vi "Timer Embedded.vi"(9 "Time Limit":u32, 10 "Reset":bool, 11 "Start Time In":u32) -> (2 "Time Limit Passed":bool, 3 "Start Time Out":u32)   [LabVIEW 2015]
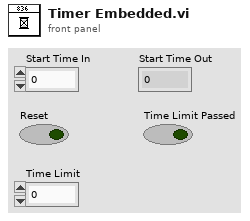
[diagram p1: front panel]
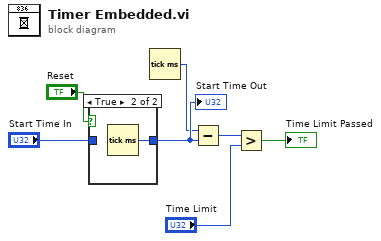
[diagram p0: block diagram]
diagram:
  n1 = case shown="True" "Reset" {
    tunnel: [w8 w9] -> w3
    tunnel: "Start Time In" -> [w8 _]
    frame False {
    }
    frame True {
      n2 = Tick Count (ms)() -> (millisecond timer value=w9:u32)
    }
  }
  "Start Time Out" <- w3
  n3 = Tick Count (ms)() -> (millisecond timer value=w2:u32)
  n4 = Subtract(x=w2, y=w3) -> (x-y=w1:u32)
  n5 = Greater?(x=w1, y="Time Limit") -> (0:→"Time Limit Passed":bool)
